vi "LCR_TrimOC.vi"(8 "error in (no error)":errorcluster, 11 "HP4284A in":refnum<class "HP4284A.lvclass">) -> (0 "error out":errorcluster, 3 "HP4284A out":refnum<class "HP4284A.lvclass">)   [LabVIEW 2018, in "HP4284A.lvclass"]
uses:
  HP4284A.lvclass
  LCRControl.lvclass
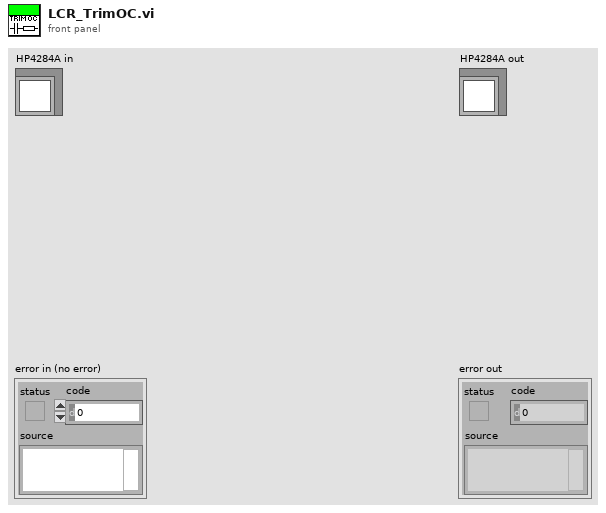
[diagram p1: front panel]
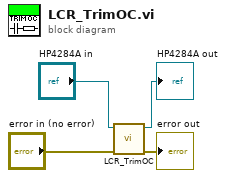
[diagram p0: block diagram]
diagram:
  n1 = call-parent "LCR_TrimOC.vi"("error in (no error)"="error in (no error)", "LCRControl in"="HP4284A in") -> ("error out"=→"error out":errorcluster, "LCRControl out"=→"HP4284A out":refnum<class "HP4284A.lvclass">)  [unwired: 8 in]
